vi "Color Cycle.vi"() -> ()   [LabVIEW 2011]
uses:
  <vilib>/Heliosphere Research LLC/Advanced Plotting Toolkit/Advanced Plotting Toolkit.lvlib
  <vilib>/Heliosphere Research LLC/Advanced Plotting Toolkit/api_annotations/LegendPositions.ctl
  <vilib>/Heliosphere Research LLC/Advanced Plotting Toolkit/properties/Marker_Style.ctl
  <vilib>/Heliosphere Research LLC/Advanced Plotting Toolkit/typedefs/PlotColor.ctl
  <vilib>/Heliosphere Research LLC/Advanced Plotting Toolkit/properties/Marker.ctl
  <vilib>/Heliosphere Research LLC/Advanced Plotting Toolkit/properties/Line_Style.ctl
  <vilib>/Heliosphere Research LLC/Advanced Plotting Toolkit/properties/Line.ctl
  <vilib>/Heliosphere Research LLC/Advanced Plotting Toolkit/properties/Colormap_Map.ctl
  <vilib>/Heliosphere Research LLC/Advanced Plotting Toolkit/properties/Colormap_Scaling.ctl
  <vilib>/Heliosphere Research LLC/Advanced Plotting Toolkit/properties/Colormap.ctl
  <vilib>/Heliosphere Research LLC/Advanced Plotting Toolkit/properties/Display.ctl
  <vilib>/Heliosphere Research LLC/Advanced Plotting Toolkit/api_plotting/ScatterProperties.ctl
panel:
  in  "Color for Set 3":T1=2147483647 items=["Automatic"=2147483647, "Black"=0, "White"=16777215, "Red"=16711680, "Green"=2263842, "Blue"=255, "Cyan"=65535, "Magenta"=16711935, "Yellow"=16776960]
  out "Color Plot":picture
  # "The Automatic Color Cycle"
  # "It's common to display multiple data sets on the same graph.\nThis is accomplished by simply calling multiple plotting VIs\nusing the same Plot ID; the data are combined onto a single\naxis automatically.\n\nIt would be tedious and error-prone to manually assign a\ndifferent color to each data set.  The Toolkit handles this\nautomatically by providing a \"color cycle\"; when making\ncalls to 1D plotting routines like Line.vi or Scatter.vi, if no\ncolor is explicitly specified, a color will be chosen automatically\nfrom a sequence of pre-defined colors.\n\nIn this example, Scatter.vi is called repeatedly to display six\ndifferent data sets.  The color of the markers is set to\n\"Automatic\" by default, which invokes the color cycle.\n\nNote that Line.vi, Scatter.vi, Bar.vi and Histogram.vi all share\nthe same color cycle for a given plot.  So if you call Scatter.vi\ntwice and then Bar.vi, the scatter points will be in blue and\ngreen, and the bar plot in red. \n\nTry changing the color for Set 3 below from \"Automatic\" to\n\"Black\".  Note that the cycle continues with the next data set."
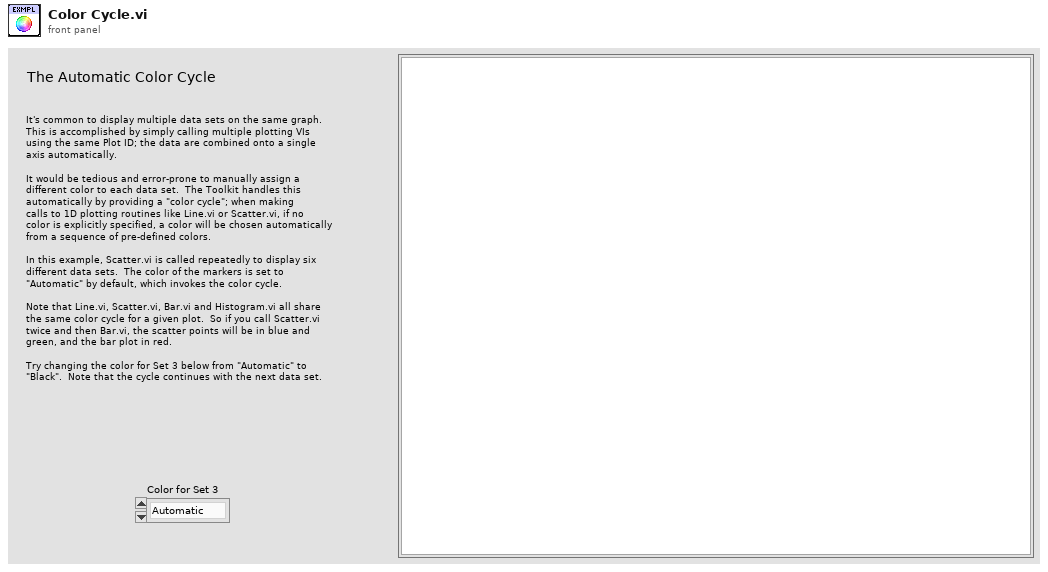
[diagram p1: front panel]
types:
  T1 = typedef "Advanced Plotting Toolkit.lvlib/PlotColor.ctl" = u32
  T2 = typedef "Advanced Plotting Toolkit.lvlib/LegendPositions.ctl" = enum16{"Default", "Top Right", "Top", "Top Left", "Left", "Bottom Left", "Bottom", "Bottom Right", "Right", "Center"}
  T3 = typedef "Advanced Plotting Toolkit.lvlib/PlotID.ctl" = i32
  T4 = typedef "Advanced Plotting Toolkit.lvlib/ScatterProperties.ctl" = cluster{"Marker":T5, "Line":T7, "Colormap":T9, "Display":T12}
  T5 = typedef "Advanced Plotting Toolkit.lvlib/Marker.ctl" = cluster{"Style":T6, "Color":T1, "Size":dbl}
  T6 = typedef "Advanced Plotting Toolkit.lvlib/Marker_Style.ctl" = enum16{"Automatic", "Circle", "Square", "Triangle", "Diamond", "Star", "Invisible"}
  T7 = typedef "Advanced Plotting Toolkit.lvlib/Line.ctl" = cluster{"Style":T8, "Color":T1, "Width":sgl}
  T8 = typedef "Advanced Plotting Toolkit.lvlib/Line_Style.ctl" = enum16{"Automatic", "Solid", "Dashed", "Dotted", "Dash-dot", "Invisible"}
  T9 = typedef "Advanced Plotting Toolkit.lvlib/Colormap.ctl" = cluster{"Map":T10, "Value Min":dbl, "Value Max":dbl, "Scaling":T11, "Reverse":bool}
  T10 = typedef "Advanced Plotting Toolkit.lvlib/Colormap_Map.ctl" = enum16{"Automatic", "Rainbow", "Hot and Cold", "White-Black", "White-Blue", "White-Green", "White-Red", "Fire", "Water", "Earth", "Air", "Pastel", "Banded", "Stepped"}
  T11 = typedef "Advanced Plotting Toolkit.lvlib/Colormap_Scaling.ctl" = enum16{"Default"}
  T12 = typedef "Advanced Plotting Toolkit.lvlib/Display.ctl" = cluster{"Alpha":dbl, "Z Order":dbl}
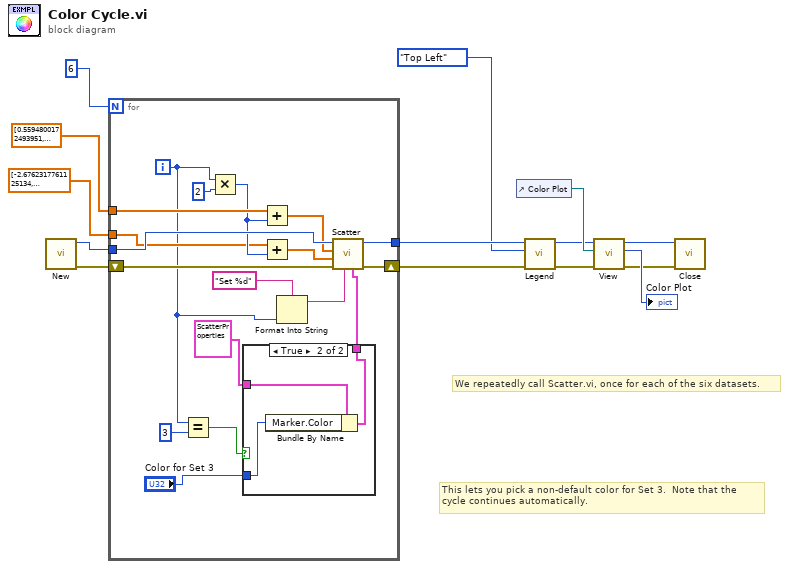
[diagram p0: block diagram]
diagram:
  # "This lets you pick a non-default color for Set 3.  Note that the\ncycle continues automatically."
  # "We repeatedly call Scatter.vi, once for each of the six datasets."
  n1 = call <vilib>:"New.vi"() -> ("error out"=w5:errorcluster, "Plot ID"=w9:T3)  [unwired: 10 in]
  n2 = for {
    N: 6 -> [_]
    tunnel: dbl[] [0.5594800172493951, 0.8354929417158985, -0.99490297010694, -0.8782976493575196, -1.121133985779089, -1.3251917000577254, 0.4843821457122872, -1.7130350835764772, 0.21747898353883974, 1.3635580896413197, 0.7585143874553933, 1.3313626878514502, -2.414298145049772, 2.2536757383752364, -0.6032899571479627, -0.41731598056307856, -0.013784647650524638, 0.10741354637861054, 0.12728478374538468, 0.9194594148239987, 0.05408153720104245, -1.2349652952195134, -0.49339182829888834, -0.1469924758888907, 1.0509212320807246, 0.26756570851731953, -0.07115202057414285, 2.1789496390336356, -2.4070431170271025, 0.4271024581543492, 0.5974963731931914, -1.9396073943190766, -1.35797979414573, 0.07989616331784861, -1.402806827303575, -0.07816487482712386, -0.05228380301527939, 1.1072423065382104, -0.5697630317112505, 0.4477881002422698, 0.16081427886943286, 1.3635651447894335, 0.7412191311973114, -0.2121069044666013, -0.14570144232903648, -0.509789786593842, -1.4692389543601305, -1.5643013917300645, 1.2326109765916702, -0.7900213854003146, 0.8008036323025733, 1.512875925048154, 1.1207302459771278, -2.5361256875470684, -1.9557133634371469, 0.11923971956997248, -0.41360678626672903, 0.19033569739228273, -0.5743230070871534, 1.2446190490155313, 1.3521941070682475, -2.930002044894795, -0.5067514813756235, -0.3321477820168344] ("Gaussian noise pattern") -> [w29]
    tunnel: dbl[] [-2.6762317761125134, -1.0709820523840066, -0.246980817582762, 0.5695150040096454, -1.7204867942492093, 0.6002650843004275, 0.5333421347622765, 0.7682184097008465, 1.2737017354242448, -0.09196711089353864, -0.6646552529384552, 0.8996518001164879, -0.5781543482415178, 0.275894601759356, -1.5829583841211547, -0.10400562044099607, 1.4953294965498785, 0.5261598608574823, 0.984721563723957, -0.7258544476951448, 1.4140124753812382, 1.9734194781711025, 1.1830494295589724, -0.9163889866946177, -0.8966365244325416, 0.9420877028649111, -2.108003778058863, -0.13224002458256578, -0.8726239040946263, -2.236746119279541, 0.34352377080084806, 0.8644013702231885, 1.1295452638287289, 0.34732642691070115, -0.15013556985218923, -0.23043345379970506, 0.3900249594961238, 0.9663691982364362, -0.1988776996664511, -0.6989570252362926, -0.6195773407074978, -0.7197990894480656, 0.5081662374633753, 0.7975968586301152, -0.36748289781266263, -0.9518793561990978, -0.08003180964734696, 1.2705204934492513, -0.2546133293618595, -0.762860826955079, -1.3793583558054183, 0.4180815914725453, 2.180254760656238, -0.9517256886330997, -0.4568074031818688, 0.4082315916138768, 0.8975563401519615, -2.304907970803578, 2.3934909675238196, 2.2067157086773257, 0.9505526515560655, -0.9752378353794683, -1.0645910085428185, 1.6062021239465167] ("Gaussian noise pattern") -> [w26]
    tunnel: w9 -> [w32]
    tunnel: [w31] -> w7
    shift-right: [w22] -> w4
    shift-left: w5 -> [w23]
    i -> [w21]
    n3 = Equal?(x=w21, y=3) -> (x = y?=w17:bool)
    n4 = Multiply(x=w21, y=2) -> (x*y=w27:i32)
    n5 = case shown="True" w17 {
      tunnel: T4 {"Marker"={"Style"=enum."Automatic", "Color"=2147483647, "Size"=nan}, "Line"={"Style"=enum."Automatic", "Color"=2147483647, "Width"=nan}, "Colormap"={"Map"=enum."Automatic", "Value Min"=nan, "Value Max"=nan, "Scaling"=enum."Default", "Reverse"=FALSE}, "Display"={"Alpha"=nan, "Z Order"=nan}} ("Scatter Properties") -> [w33 w36]
      tunnel: [w33 w35] -> w18
      tunnel: "Color for Set 3" -> [_ w34]
      frame False {
      }
      frame True {
        n6 = Bundle By Name(cluster=w36, "Marker.Color"=w34) -> (w35:T4)
      }
    }
    n7 = Add(x=w29, y=w27) -> (x+y=w28:dbl[])
    n8 = Add(x=w26, y=w27) -> (x+y=w25:dbl[])
    n9 = Format Into String(format string="Set %d", w21) -> (resulting string=w15:string)  [unwired: 2 in, 1 out]
    n10 = call <vilib>:"Scatter.vi"("Properties"=w18, "Legend Title"=w15, "error in (no error)"=w23, "Y Data"=w25, "X Data"=w28, "Plot ID"=w32) -> ("error out"=w22:errorcluster, "Plot ID Out"=w31:T3)  [unwired: 4 in]
  }
  n11 = control-ref of="Color Plot"() -> (w14:refnum<vi>)
  n12 = call <vilib>:"Legend.vi"("error in (no error)"=w4, "Position"=LegendPositions."Top Left", "Plot ID"=w7) -> ("error out"=w3:errorcluster, "Plot ID Out"=w6:T3)  [unwired: 7 in]
  n13 = call <vilib>:"View.vi"("error in (no error)"=w3, "Ref for Sizing"=w14, "Plot ID"=w6) -> ("error out"=w1:errorcluster, "Picture"=→"Color Plot":picture, "Plot ID Out"=w12:T3)  [unwired: 6 in]
  n14 = call <vilib>:"Close.vi"("error in (no error)"=w1, "Plot ID"=w12) -> ()  [unwired: 9 in, 1 out]
